vi "HTML_Header_Include_CreateTagElement.vi"(5 "HTML-Tag-Type":T1=enum."JS-Tag", 7 "rel links (f) / include in .html (T)":bool, 8 "Error In":errorcluster, 9 "rel. Filepaths .css":path[](array[path]), 10 "abs Path to files on disk":path, 11 "relative Path to ContentFolder":path) -> (0 "Error Out":errorcluster, 1 "<head> String (Out)":string, 2 "<head> tags[] (Out)":string[](array[string]))   [LabVIEW 2014]
uses:
  controls/HTML_Tag_Type.ctl
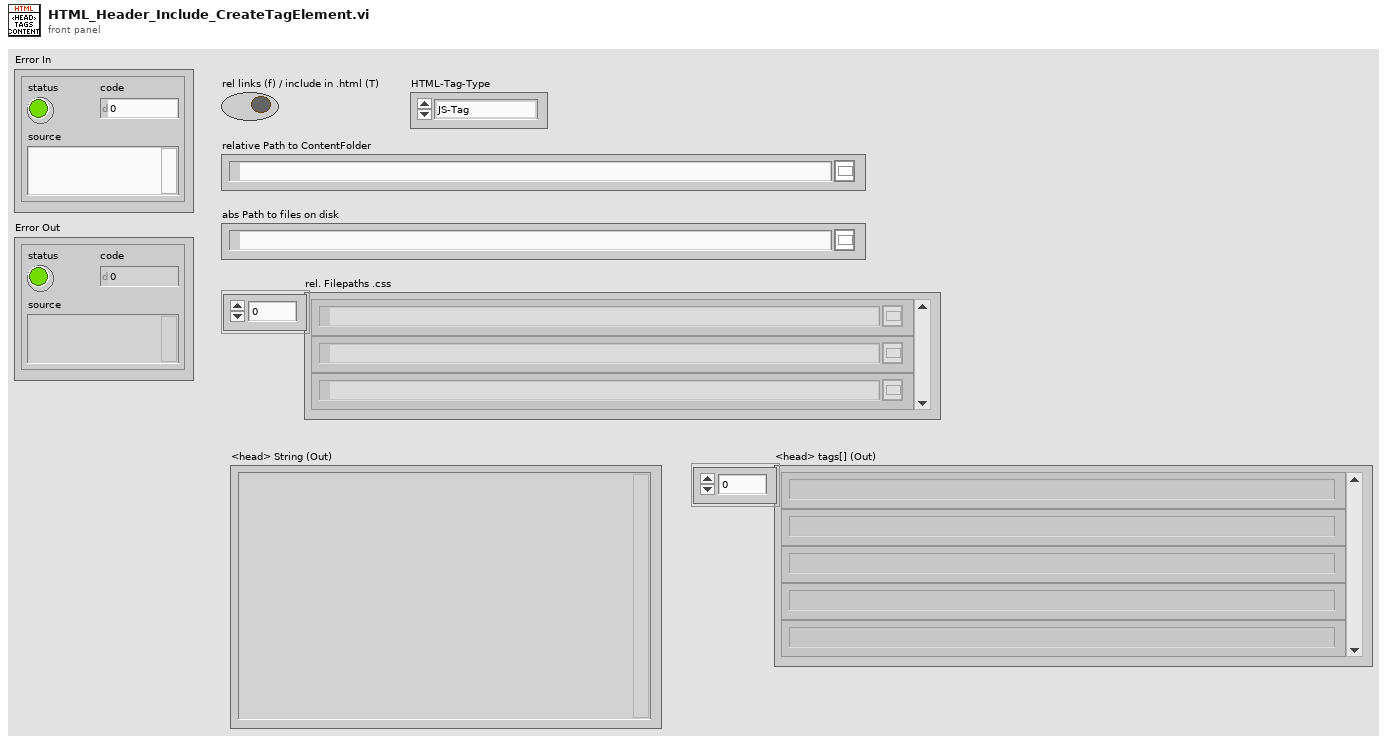
[diagram p1: front panel]
types:
  T1 = typedef "HTML_Tag_Type.ctl" = enum16{"CSS-Tag", "JS-Tag"}
  T2 = enum16{"open", "replace", "create", "open or create", "replace or create", "replace or create with confirmation"}
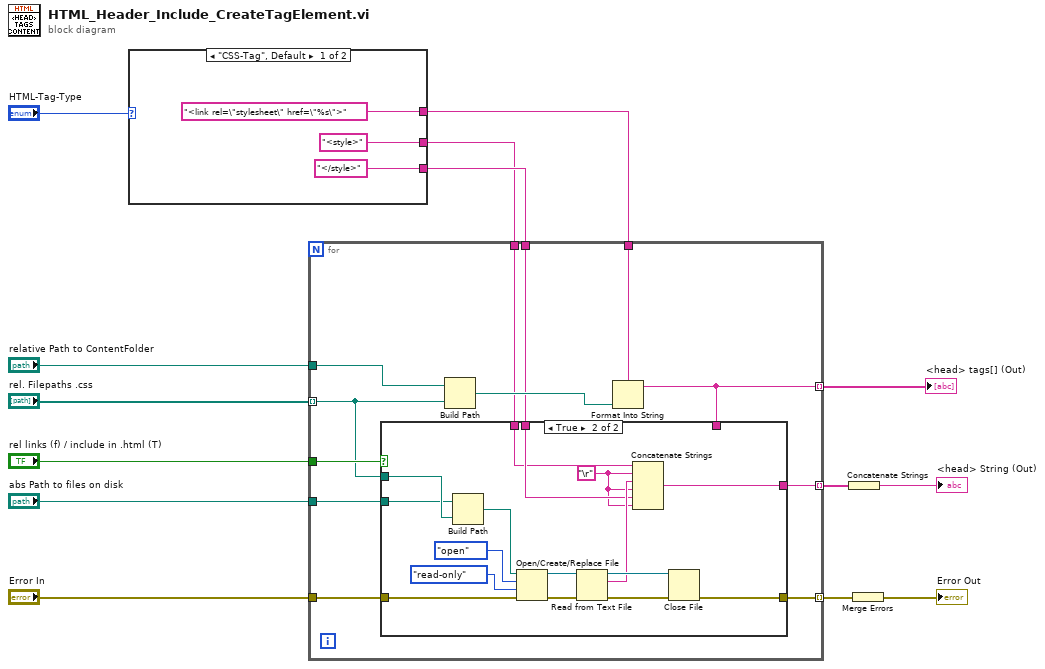
[diagram p0: block diagram]
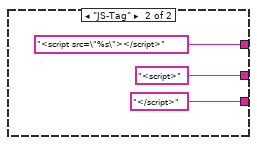
[diagram p2: hidden frame]
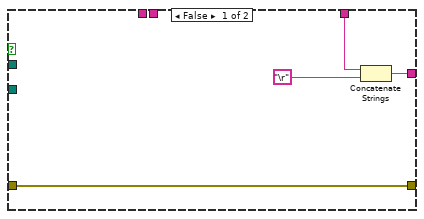
[diagram p3: hidden frame]
diagram:
  n1 = case shown="\"CSS-Tag\", Default" "HTML-Tag-Type" {
    tunnel: ["<link rel=\"stylesheet\" href=\"%s\">" ("format string") "<script src=\"%s\"></script>" ("format string")] -> w3
    tunnel: ["</style>" ("format string") "</script>" ("format string")] -> w2
    tunnel: ["<style>" ("format string") "<script>" ("format string")] -> w1
    frame "CSS-Tag", Default {
    }
    frame "JS-Tag" {
    }
  }
  n2 = for {
    tunnel: [w31] -> w11 mode=indexing
    tunnel: "rel. Filepaths .css" -> [w24] mode=indexing
    tunnel: "relative Path to ContentFolder" -> [w25]
    tunnel: [w30] -> w12 mode=indexing
    tunnel: "abs Path to files on disk" -> [w29]
    tunnel: "rel links (f) / include in .html (T)" -> [w28]
    tunnel: "Error In" -> [w27]
    tunnel: [w26] -> w6 mode=indexing
    tunnel: w3 -> [w23]
    tunnel: w1 -> [w22]
    tunnel: w2 -> [w21]
    n3 = Build Path(base path=w25, name or relative path=w24) -> (appended path=w32:path)
    n4 = Format Into String(format string=w23, w32) -> (resulting string=w31:string)  [unwired: 2 in, 1 out]
    n5 = case shown="True" w28 {
      tunnel: w31 -> [w36 _]
      tunnel: [w34 w46] -> w30
      tunnel: w29 -> [_ w43]
      tunnel: w27 -> [w33 w47]
      tunnel: [w33 w48] -> w26
      tunnel: w24 -> [_ w44]
      tunnel: w21 -> [_ w39]
      tunnel: w22 -> [_ w38]
      frame False {
        n6 = Concatenate Strings(w36, "\r") -> (w34:string)
      }
      frame True {
        w37 = "\r"
        n7 = Build Path(base path=w43, name or relative path=w44) -> (appended path=w42:path)
        n8 = Open/Create/Replace File(file path (use dialog)=w42, error in=w47, operation (0:open)=T2."open", access (0:read/write)=enum16{"read/write", "read-only", "write-only"}."read-only") -> (refnum out=w49:refnum<file>, error out=w50:errorcluster)  [unwired: 2 in, 1 out]
        n9 = Read from Text File(file (use dialog)=w49, error in=w50) -> (refnum out=w51:refnum<file>, text=w45:string, error out=w52:errorcluster)  [unwired: 2 in, 1 out]
        n10 = Concatenate Strings(w38, w37, w45, w37, w39, w37) -> (w46:string)
        n11 = Close File(refnum=w51, error in=w52) -> (error out=w48:errorcluster)  [unwired: 1 out]
      }
    }
  }
  "<head> tags[] (Out)" <- w11
  n12 = Concatenate Strings(w12) -> (→"<head> String (Out)":string)
  n13 = Merge Errors(w6) -> (→"Error Out":errorcluster)
